vi "Get Code Generation Information.vi"(8 "error in (no error)":errorcluster, 11 "RIO Target in":refnum<class "RIO Target.lvclass">) -> (0 "error out":errorcluster, 2 "Bus Information Array":T1[](array[typedef]), 3 "RIO Target out":refnum<class "RIO Target.lvclass">)   [LabVIEW 2014, in "RIO Target.lvclass"]
uses:
  RIO Target.lvclass
  Scripting/Initialization Scripting/State Machine/Controls/Bus Information.ctl
  Scripting/Initialization Scripting/State Machine/Controls/Device Information.ctl
  Scripting/Initialization Scripting/State Machine/Controls/Pin Information.ctl
  <vilib>/NI/Configuration Framework/Node/NISE_CEF_Node.lvclass/NISE_CEF_Node.ctl
  Bus/Bus.lvclass
  Bus Configuration/Bus Configuration.lvclass
  Bus Configuration/Bus Configuration.lvclass/Bus Configuration.ctl
  <vilib>/NI/Configuration Framework/Node/NISE_CEF_Node.lvclass
  <vilib>/NI/Configuration Framework/serializable configuration/NISE_CEF_serializable configuration.lvclass
  Scripting/Initialization Scripting/Initialization and IO Node Scripting.lvlib
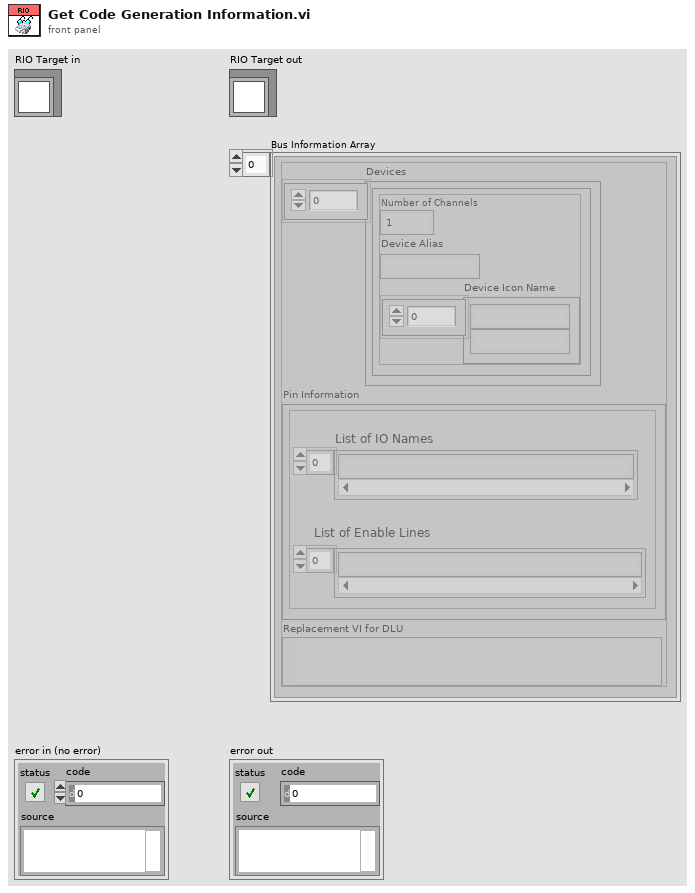
[diagram p1: front panel]
types:
  T1 = typedef "Initialization and IO Node Scripting.lvlib/Bus Information.ctl" = cluster{"Devices":T2[], "Pin Information":T3, "Replacement VI for DLU":path}
  T2 = typedef "Device Information.ctl" = cluster{"Number of Channels":i32, "Device Alias":string, "Device Icon Name":string[]}
  T3 = typedef "Pin Information.ctl" = cluster{"List of IO Names":string[], "List of Enable Lines":string[]}
  T4 = typedef "NISE_CEF_Node.lvclass/NodeRef.ctl" = refnum<data-value>
  T5 = typedef "Bus Configuration.lvclass/SPI Configuration.ctl" = cluster{"SCLK":string, "MOSI":string, "MISO":string}
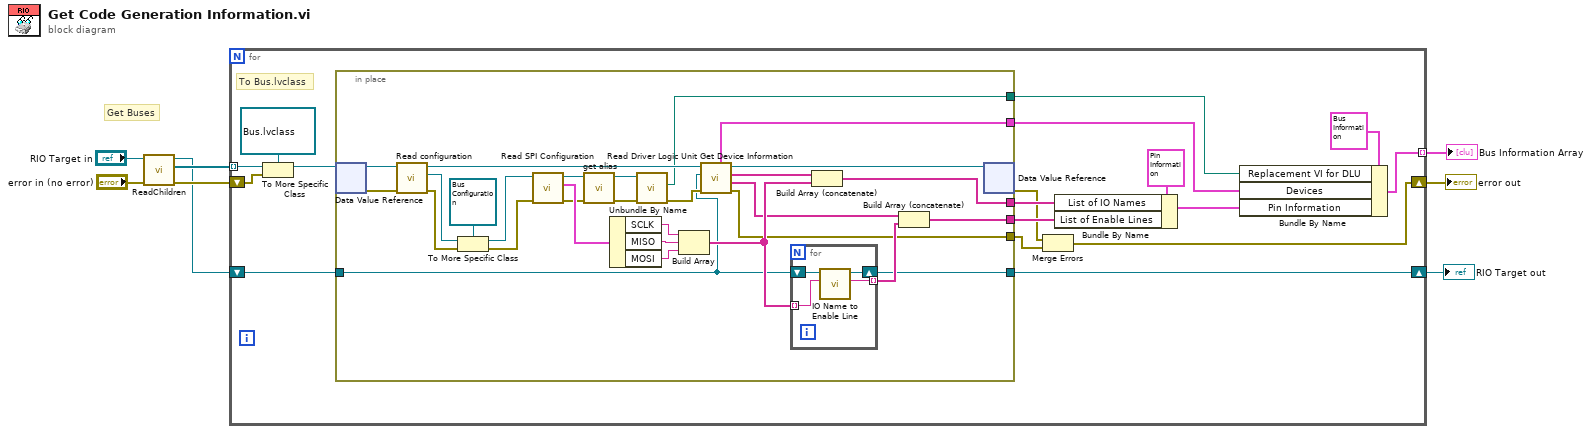
[diagram p0: block diagram]
diagram:
  # "Get Buses"
  n1 = call <vilib>:"ReadChildren.vi"("error in"="error in (no error)", "node in"="RIO Target in") -> ("error out"=w3:errorcluster, "output array"=w5:T4[], "node out"=w2:refnum<class "RIO Target.lvclass">)  [unwired: 7 in]
  n2 = for {
    tunnel: w5 -> [w25] mode=indexing
    shift-right: [w11] -> w8
    shift-left: w3 -> [w22]
    tunnel: [w21] -> w7 mode=indexing
    shift-right: [w9] -> w1
    shift-left: w2 -> [w17]
    # "To Bus.lvclass"
    n3 = To More Specific Class(target class=refnum<data-value> refnum ("data value reference"), reference=w25, error in=w22) -> (specific class reference=w23:refnum<data-value>)  [unwired: 1 out]
    n4 = in-place {
      in-place-border: w17 -> [w26]
      in-place-border: [w33] -> w16
      in-place-border: [w32] -> w15
      in-place-border: [w31] -> w14
      in-place-border: [w29] -> w13
      in-place-border: [w28] -> w10
      in-place-border: [w27] -> w9
      n5 = in-place-dvr #1(w23) -> (w54:refnum<class "Bus.lvclass">, w47:errorcluster)
      n6 = call-dynamic "Read configuration.vi"("error in"=w47, "Bus in"=w54) -> ("error out"=w46:errorcluster, "configuration"=w53:refnum<class "NISE_CEF_serializable configuration.lvclass">, "Bus out"=w45:refnum<class "Bus.lvclass">)  [unwired: 7 in]
      n7 = To More Specific Class(target class=refnum<class "Bus Configuration.lvclass"> refnum ("Bus Configuration.lvclass"), reference=w53, error in=w46) -> (specific class reference=w51:refnum<class "Bus Configuration.lvclass">, error out=w44:errorcluster)
      n8 = call "Read SPI Configuration.vi"("error in (no error)"=w44, "Bus Configuration in"=w51) -> ("error out"=w43:errorcluster, "SPI Configuration"=w49:T5, "Bus Configuration out"=w50:refnum<class "Bus Configuration.lvclass">)  [unwired: 7 in]
      n9 = call <vilib>:"get alias.vi"("error in"=w43, "configuration in"=w50) -> ("error out"=w42:errorcluster, "configuration out"=w48:refnum<class "Bus Configuration.lvclass">)  [unwired: 7 in, 1 out]
      n10 = Unbundle By Name(w49) -> ("SCLK"=w41:string, "MISO"=w40:string, "MOSI"=w39:string)
      n11 = call "Read Driver Logic Unit.vi"("error in (no error)"=w42, "Bus Configuration in"=w48) -> ("error out"=w30:errorcluster, "Driver Logic Unit"=w28:path)  [unwired: 7 in, 1 out]
      n12 = Build Array(w41, w40, w39) -> (w37:string[])
      n13 = call "Get Device Information.vi"("error in"=w30, "RIO Target in"=w26, "Bus in"=w45) -> ("error out"=w29:errorcluster, "Enable Lines"=w35:string[], "Chip Select Lines"=w38:string[], "Bus out"=w34:refnum<class "Bus.lvclass">, "Device Information Array"=w31:T2[])  [unwired: 4 in]
      n14 = for {
        shift-right: [w57] -> w27
        shift-left: w26 -> [w58]
        tunnel: [w56] -> w36 mode=indexing
        tunnel: w37 -> [w55] mode=indexing
        n15 = call-dynamic "IO Name to Enable Line.vi"("IO Name"=w55, "RIO Target in"=w58) -> ("Enable Line"=w56:string, "RIO Target out"=w57:refnum<class "RIO Target.lvclass">)  [unwired: 7 in, 1 out]
      }
      n16 = Build Array (concatenate)(w38, w37) -> (w33:string[])
      n17 = Build Array (concatenate)(w35, w36) -> (w32:string[])
      n18 = in-place-dvr #1(w34) -> (w12:errorcluster)  [unwired: 1 out]
    }
    n19 = Merge Errors(w12, w13) -> (w11:errorcluster)
    n20 = Bundle By Name(cluster=T3 {"List of IO Names"=["sbRIO-9651 Socket\\PMOD1_Pin4_out", "sbRIO-9651 Socket\\PMOD1_Pin3_in", "sbRIO-9651 Socket\\PMOD1_Pin2_out", "sbRIO-9651 Socket\\PMOD1_Pin1_out"], "List of Enable Lines"=["sbRIO-9651 Socket\\PMOD1_Pin4_enable", "sbRIO-9651 Socket\\PMOD1_Pin3_enable", "sbRIO-9651 Socket\\PMOD1_Pin2_enable", "sbRIO-9651 Socket\\PMOD1_Pin1_enable"]} ("Pin Information"), "List of IO Names"=w16, "List of Enable Lines"=w15) -> (w18:T3)
    n21 = Bundle By Name(cluster=T1 {"Devices"=[], "Pin Information"={"List of IO Names"=["sbRIO-9651 Socket\\PMOD1_Pin4_out", "sbRIO-9651 Socket\\PMOD1_Pin3_in", "sbRIO-9651 Socket\\PMOD1_Pin2_out", "sbRIO-9651 Socket\\PMOD1_Pin1_out"], "List of Enable Lines"=["sbRIO-9651 Socket\\PMOD1_Pin4_enable", "sbRIO-9651 Socket\\PMOD1_Pin3_enable", "sbRIO-9651 Socket\\PMOD1_Pin2_enable", "sbRIO-9651 Socket\\PMOD1_Pin1_enable"]}, "Replacement VI for DLU"=path "E:/Documents/Projects/SPIAPI/Scripting Code  with State Machine 01_16_15 - Integrating with GUI/Test/Replacement.vi"} ("Bus Information"), "Replacement VI for DLU"=w10, "Devices"=w14, "Pin Information"=w18) -> (w21:T1)
  }
  "error out" <- w8
  "RIO Target out" <- w1
  "Bus Information Array" <- w7
